vi "ATF-Storage-DI SEQ MAIN.vi"(8 "error in":errorcluster) -> (0 "error Out":errorcluster)   [LabVIEW 2022 SP3]
uses:
  RT Controls/ATF Storage-FGV Read write.ctl
  <vilib>/platform/TimedLoop/XDataNode/XDataNode.xnode
  <vilib>/Platform/TimedLoop/XDataNode/nitl_modes.ctl
  <vilib>/Platform/TimedLoop/XDataNode/XDNodeRunTimeDep.lvlib
  <vilib>/Platform/TimedLoop/XDataNode/wakeup.ctl
  <vilib>/Platform/TimedLoop/XDataNode/timing_clust.ctl
panel:
  out "Failure \ncase Seq":string[](array[string])
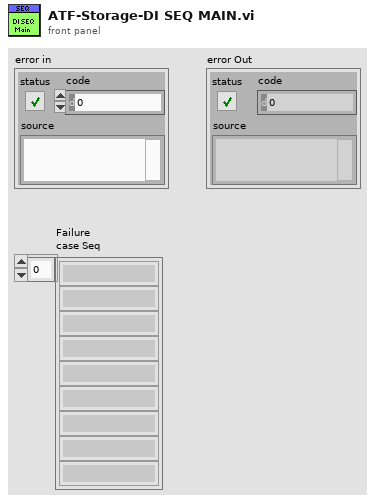
[diagram p1: front panel]
types:
  T1 = typedef "XDNodeRunTimeDep.lvlib/timing_clust.ctl" = cluster{"Expected End [f-1]":u64, "Actual End [f-1]":u64, "Finished Late? [f-1]":bool, "Expected End [i-1]":u64, "Actual End [i-1]":u64, "Finished Late? [i-1]":bool, "Expected Start [i]":u64, "Actual Start [i]":u64, "Expected Start [f]":u64, "Actual Start [f]":u64, "Source Name":string, "Structure Name":string, "Period":i64, "Deadline":i64, "Offset":i64, "Start":i64, "Priority":i32, "Timeout":i32, "Mode":T2, "Wakeup Reason":T3, "Error":errorcluster, "Source Type":string, "Secondary Source Type":string, "Global End Time":u64, "Global Start Time":u64, "Frame Duration":u64, "Iteration Duration":u64, "Assigned CPU":i32, "I/O Scan Engine Mode":u32}
  T2 = typedef "XDNodeRunTimeDep.lvlib/nitl_modes.ctl" = enum32{"No Change", "Process missed periods, maintain original phase", "Discard missed periods, maintain original phase", "Process missed periods, ignore original phase", "Discard missed periods, ignore original phase"}
  T3 = typedef "XDNodeRunTimeDep.lvlib/wakeup.ctl" = enum32{"Normal", "Aborted", "Asynchronous wakeup", "Timing source error", "Timed loop error", "Timeout"}
  T4 = typedef "ATF Storage-FGV Read write.ctl" = enum16{"Write", "Read"}
  T5 = cluster{"Manual HOLD":bool, "Automatic Hold AI":bool, "Abort":bool, "Automatic Hold DI":bool}
  T6 = cluster{"Start DAQ":bool, "Stop DAQ":bool, "RT Stop":bool, "RT Exit":bool, "Start Seq":bool}
  T7 = cluster{cluster{"Sr. No.":string, "Time CDT":string, "Component ID":string, "Data Type":string, "Condition":string, "Range/Position":string, "No of Samples for Pass":string, "Event Duration":string, "Continuous /Cumulative":string, "Expected Delay":string, "Failure case Seq":string, "Current Sequence":string}[]}[]
  T8 = cluster{cluster{"Sr. No.":string, "Time CDT":string, "Component ID":string, "Data Type":string, "Condition":string, "Range/Position":string, "No of Samples for Pass":string, "Event Duration":string, "Continuous /Cumulative":string, "Expected Delay":string, "Failure case Seq":string, "Current Sequence":string}[]}
  T9 = cluster{"Sr. No.":string, "Time CDT":string, "Component ID":string, "Data Type":string, "Condition":string, "Range/Position":string, "No of Samples for Pass":string, "Event Duration":string, "Continuous /Cumulative":string, "Expected Delay":string, "Failure case Seq":string, "Current Sequence":string}[]
  T10 = cluster{"Sr. No.":string, "Time CDT":string, "Component ID":string, "Data Type":string, "Condition":string, "Range/Position":string, "No of Samples for Pass":string, "Event Duration":string, "Continuous /Cumulative":string, "Expected Delay":string, "Failure case Seq":string, "Current Sequence":string}
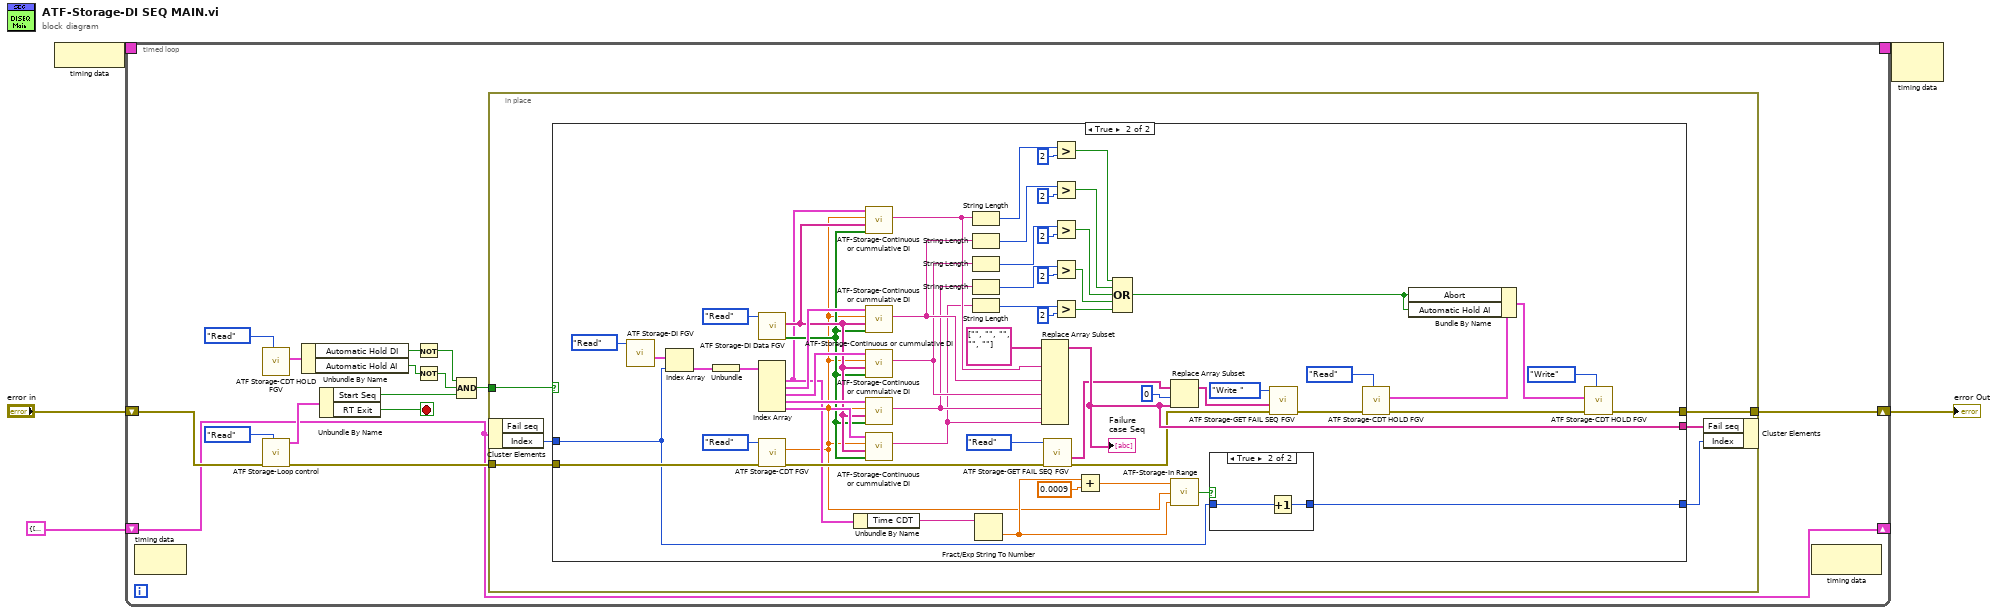
[diagram p0: block diagram]
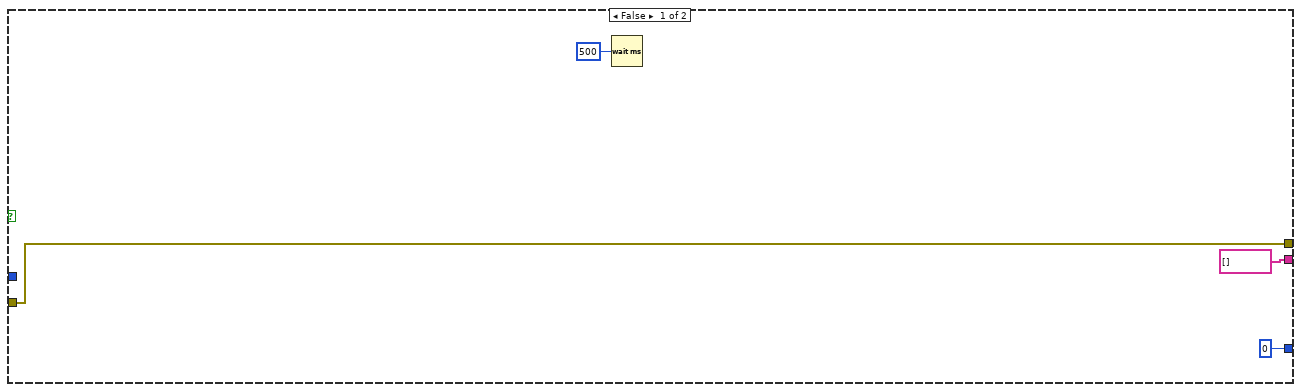
[diagram p2: hidden frame]
diagram:
  n1 = node-c288() -> (w3:T1)
  n2 = timed-loop {
    shift-right: [w15] -> w5
    shift-left: "error in" -> [w18]
    timing: w3 -> [_]
    timing-out: [_] -> w2
    shift-right: [w6] -> _
    shift-left: cluster{"Fail seq":string[], "Index":i32} {"Fail seq"=["", "", "", "", ""], "Index"=0} -> [w6]
    stop <- w16 stop-if-true
    n3 = node-c288() -> ()  [unwired: 1 in, 1 out]
    n4 = call "ATF Storage-CDT HOLD FGV.vi"("Write/Read"=enum16{"Write", "Read"}."Read") -> ("HOLD and Abort Out"=w8:T5)  [unwired: 7 in, 1 out]
    n5 = call "ATF Storage-Loop control.vi"("Action"=enum16{"Init", "Write", "Read"}."Read", "error in (no error)"=w18) -> ("error Out"=w17:errorcluster, "Loop Control out"=w19:T6)  [unwired: 8 in]
    n6 = Unbundle By Name(w8) -> ("Automatic Hold DI"=w10:bool, "Automatic Hold AI"=w12:bool)
    n7 = Unbundle By Name(w19) -> ("Start Seq"=w7:bool, "RT Exit"=w16:bool)
    n8 = Not(x=w10) -> (.not. x?=w9:bool)
    n9 = Not(x=w12) -> (.not. x?=w13:bool)
    n10 = Compound Arithmetic op=AND(w9, w13, w7) -> (w11:bool)
    n11 = in-place "In Place Element Structure" {
      in-place-border: w17 -> [w26]
      in-place-border: [w25] -> w15
      in-place-border: w11 -> [w24]
      n12 = in-place-cluster #1(w6) -> ("Index"=w22:i32)  [unwired: 1 out]
      n13 = case shown="True" w24 {
        tunnel: w26 -> [w30 w89]
        tunnel: [w30 w86] -> w25
        tunnel: [0 ("Index") w85] -> w23
        tunnel: w22 -> [_ w32]
        tunnel: [string[] [] ("Fail seq") w84] -> w21
        frame False {
          n14 = Wait (ms)(milliseconds to wait=u32 500) -> ()  [unwired: 1 out]
        }
        frame True {
          n15 = call "ATF Storage-DI FGV.vi"("Enum"=enum16{"Read", "Write "}."Read") -> ("DI Seq  OUT"=w34:T7)  [unwired: 9 in, 1 out]
          n16 = Index Array(array=w34, index=w32) -> (element=w33:T8)
          n17 = Unbundle(w33) -> (w78:T9)
          n18 = call "ATF Storage-DI Data FGV.vi"("Write/Read"=ATF_Storage-FGV_Read_write."Read") -> ("DI Y LP"=w75:bool[], "DI Signal List LP"=w76:string[])  [unwired: 8 in, 1 out]
          n19 = Index Array(array=w78) -> (element #1=w37:T10, element #2=w82:T10, element #3=w81:T10, element #4=w80:T10, element #5=w79:T10)  [unwired: 5 in]
          n20 = call "ATF Storage-CDT FGV.vi"("error in (no error)"=w89, "Write/Read"=enum16{"Write", "Read"}."Read") -> ("error Out"=w69:errorcluster, "CDT Out"=w31:dbl)  [unwired: 8 in]
          n21 = Unbundle By Name(w37) -> ("Time CDT"=w36:string)
          n22 = call "ATF-Storage-Continuous or cummulative DI.vi"("DI   data"=w75, "DI Channels Name"=w76, "CDT"=w31, "output cluster"=w37) -> ("Failure case Seq"=w57:string)  [unwired: 6 in, 1 out]
          n23 = call "ATF-Storage-Continuous or cummulative DI.vi"("DI   data"=w75, "DI Channels Name"=w76, "CDT"=w31, "output cluster"=w82) -> ("Failure case Seq"=w56:string)  [unwired: 6 in, 1 out]
          n24 = call "ATF-Storage-Continuous or cummulative DI.vi"("DI   data"=w75, "DI Channels Name"=w76, "CDT"=w31, "output cluster"=w81) -> ("Failure case Seq"=w55:string)  [unwired: 6 in, 1 out]
          n25 = call "ATF-Storage-Continuous or cummulative DI.vi"("DI   data"=w75, "DI Channels Name"=w76, "CDT"=w31, "output cluster"=w80) -> ("Failure case Seq"=w54:string)  [unwired: 6 in, 1 out]
          n26 = call "ATF-Storage-Continuous or cummulative DI.vi"("DI   data"=w75, "DI Channels Name"=w76, "CDT"=w31, "output cluster"=w79) -> ("Failure case Seq"=w53:string)  [unwired: 6 in, 1 out]
          n27 = String Length(string=w57) -> (length=w62:i32)
          n28 = String Length(string=w56) -> (length=w61:i32)
          n29 = String Length(string=w55) -> (length=w60:i32)
          n30 = String Length(string=w54) -> (length=w59:i32)
          n31 = String Length(string=w53) -> (length=w58:i32)
          n32 = Fract/Exp String To Number(string=w36) -> (number=w35:dbl)  [unwired: 3 in, 1 out]
          n33 = Replace Array Subset(array=string[] ["", "", "", "", ""], new element #1=w57, new element #2=w56, new element #3=w55, new element #4=w54, new element #5=w53) -> (w84:string[])  [unwired: 5 in]
          "Failure \ncase Seq" <- w84
          n34 = call "ATF Storage-GET FAIL SEQ FGV.vi"("error in"=w69, "Enum"=enum16{"Read", "Write "}."Read") -> ("error out"=w68:errorcluster, "Failure \ncase Seq"=w72:string[])  [unwired: 8 in]
          n35 = Greater?(x=w62, y=2) -> (0:w52:bool)
          n36 = Greater?(x=w61, y=2) -> (0:w51:bool)
          n37 = Greater?(x=w60, y=2) -> (0:w50:bool)
          n38 = Greater?(x=w59, y=2) -> (0:w49:bool)
          n39 = Greater?(x=w58, y=2) -> (0:w48:bool)
          n40 = Add(x=w35, y=0.0009) -> (x+y=w40:dbl)
          n41 = Compound Arithmetic op=OR(w52, w51, w50, w49, w48) -> (w41:bool)
          n42 = Replace Array Subset(array=w72, new element=w84, index=0) -> (w70:string[])
          n43 = call "ATF-Storage-In Range.vi"("Min"=w35, "X"=w31, "Max"=w40) -> ("In Range"=w38:bool)  [unwired: 2 in]
          n44 = case shown="True" w38 {
            tunnel: w32 -> [w90 w92]
            tunnel: [w90 w91] -> w85
            frame False {
            }
            frame True {
              n45 = Increment(x=w92) -> (x+1=w91:i32)
            }
          }
          n46 = call "ATF Storage-GET FAIL SEQ FGV.vi"("error in"=w68, "Failure \ncase Seq"=w70, "Enum"=enum16{"Read", "Write "}."Write ") -> ("error out"=w42:errorcluster)  [unwired: 7 in, 1 out]
          n47 = call "ATF Storage-CDT HOLD FGV.vi"("Write/Read"=enum16{"Write", "Read"}."Read", "error in (no error)"=w42) -> ("error Out"=w45:errorcluster, "HOLD and Abort Out"=w44:T5)  [unwired: 6 in]
          n48 = Bundle By Name(cluster=w44, "Abort"=w41, "Automatic Hold AI"=w41) -> (w43:T5)
          n49 = call "ATF Storage-CDT HOLD FGV.vi"("Write/Read"=enum16{"Write", "Read"}."Write", "error in (no error)"=w45, "HOLD and Abort"=w43) -> ("error Out"=w86:errorcluster)  [unwired: 5 in, 1 out]
        }
      }
      n50 = in-place-cluster #1("Fail seq"=w21, "Index"=w23) -> ()  [unwired: 1 out]
    }
    n51 = node-c288() -> ()  [unwired: 1 in, 1 out]
  }
  "error Out" <- w5
  n52 = node-c288(w2) -> ()  [unwired: 1 out]
